vi "Sensor_Readings_Intg.vi"(0 "LINX Resource in":T1, 1 "Gyro Offset Y":i16, 2 "Gyro Offset X":i16, 3 "I2C Slave Address":T7, 4 "Milliseconds to wait in":u32=1, 5 "Acc Offset X":dbl[](array[numeric])=[30.0], 6 "Acc Offset Y":dbl[](array[numeric])=[90.0], 7 "error in (no error)":errorcluster) -> (20 "LINX Resource out":T1, 21 "Gyro Angle X":dbl(graph), 22 "Gyro Angle Y":dbl(graph), 23 "Milliseconds to wait out":u32=1, 24 "Acc Angle X":dbl[](graph)=[-22.25165725221299], 25 "Acc Angle Y":dbl[](graph)=[-0.6417100508007536], 27 "error out":errorcluster)   [LabVIEW 2021]
uses:
  <vilib>/MakerHub/LINX/Private/Type Defs/LINX Ref.ctl
  <vilib>/MakerHub/LINX/Private/Type Defs/Platform.ctl
  <vilib>/MakerHub/LINX/Private/Type Defs/Interface.ctl
  <vilib>/MakerHub/LINX/Private/Device/Type Defs/LINX Device Config.ctl
  <vilib>/MakerHub/LINX/Private/Device/Type Defs/TCP Config.ctl
  <vilib>/MakerHub/LINX/Private/Device/Type Defs/Channels.ctl
  <vilib>/MakerHub/LINX/Public/Sensors/Accelerometer/MPU60X0/DeviceAddresses.ctl
  <vilib>/MakerHub/LINX/Public/Sensors/Accelerometer/MPU60X0/MPU60X0.lvlib
  <vilib>/MakerHub/LINX/LMH-LINX.lvlib
  <vilib>/MakerHub/LINX/Private/Device/Device.lvlib
panel:
  out "Acceleration Graph":T8(graph)={"X Axis"=-7900, "Y Axis"=-136, "Z Axis"=-14032}
  out "Acceleration Data (g)":T8={"X Axis"=-7900, "Y Axis"=-136, "Z Axis"=-14032}
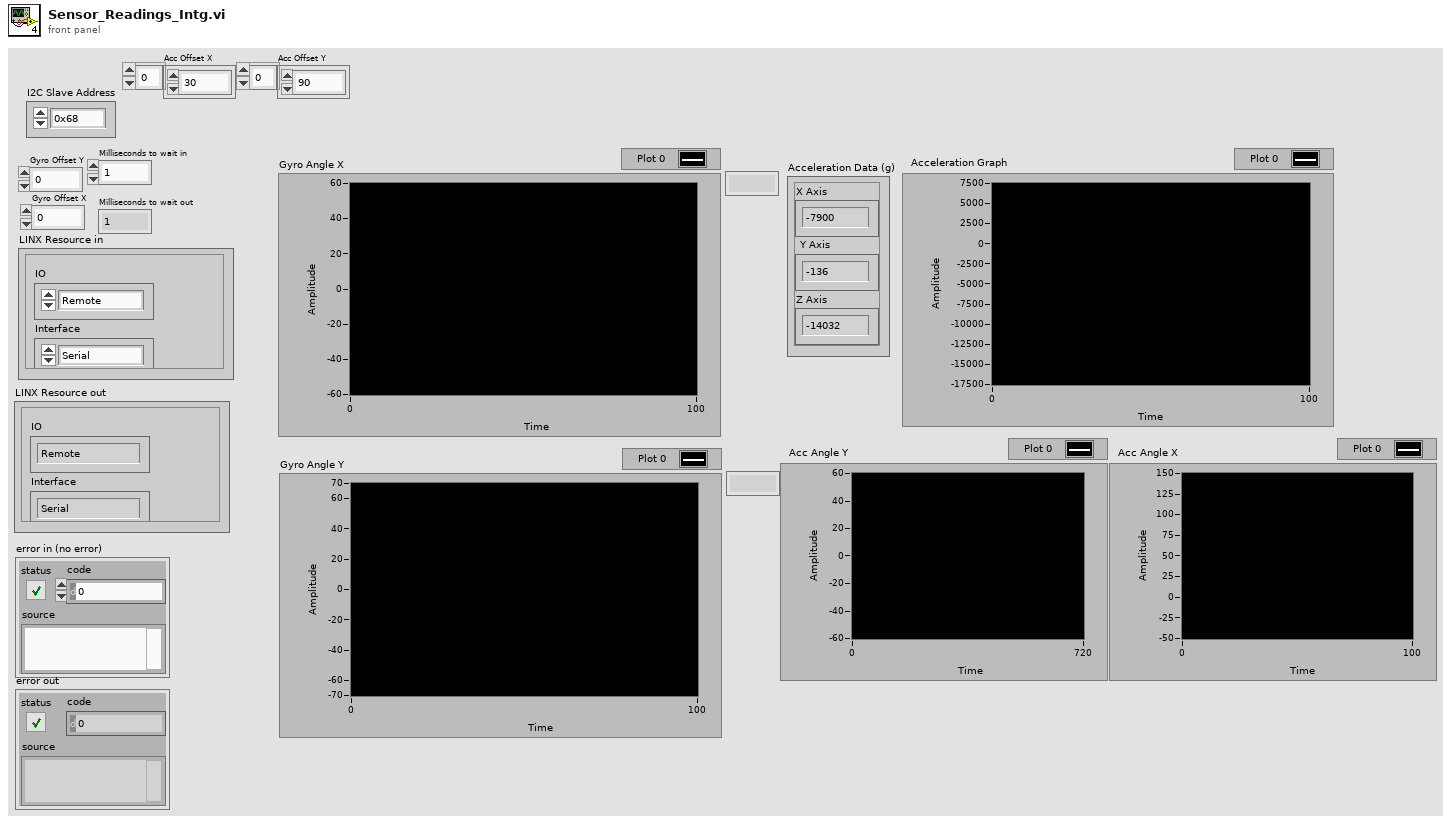
[diagram p1: front panel]
types:
  T1 = typedef "LMH-LINX.lvlib/LINX Ref.ctl" = cluster{"IO":T2, "Interface":T3, "LINX Device Config":T4}
  T2 = typedef "LMH-LINX.lvlib/Platform.ctl" = enum16{"Remote", "Local"}
  T3 = typedef "LMH-LINX.lvlib/Interface.ctl" = enum16{"Serial", "TCP"}
  T4 = typedef "LMH-LINX.lvlib/Device.lvlib/LINX Device Config.ctl" = cluster{"Interface":T3, "COM Port":refnum<visa-resource-name>, "TCP Configuration":T5, "Device Family":u8, "Device ID":u8, "Device Name":string, "TCP Ref":refnum<k5>, "Channels":T6}
  T5 = typedef "LMH-LINX.lvlib/Device.lvlib/TCP Config.ctl" = cluster{"IP Address":string, "Port":u16}
  T6 = typedef "LMH-LINX.lvlib/Channels.ctl" = cluster{"DI":u8[], "DO":u8[], "AI":u8[], "AO":u8[], "PWM":u8[], "QE":u8[], "UART":u8[], "I2C 2":u8[], "SPI":u8[], "CAN":u8[], "Servo":u8[], "AI Ref (V)":dbl, "AI Resolution (Bits)":u8, "AO Ref (V)":dbl, "AO Resolution (Bits)":u8}
  T7 = typedef "LMH-LINX.lvlib/MPU60X0.lvlib/DeviceAddresses.ctl" = enum16{"0x68", "0x69"}
  T8 = cluster{"X Axis":i16, "Y Axis":i16, "Z Axis":i16}
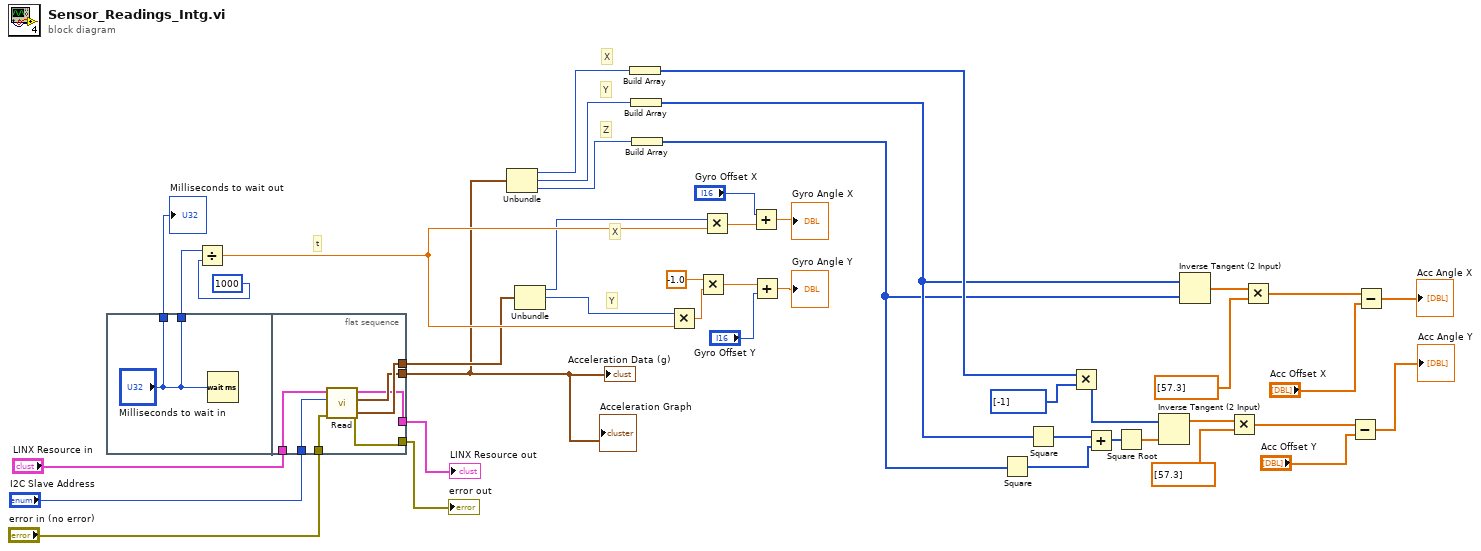
[diagram p0: block diagram]
diagram:
  # "Z"
  # "Y"
  # "X"
  # "X"
  # "Y"
  # "t"
  n1 = flat-sequence {
    tunnel: ["Milliseconds to wait in"] -> w41
    tunnel: ["Milliseconds to wait in"] -> w25
    tunnel: "error in (no error)" -> [w51]
    tunnel: "LINX Resource in" -> [w50]
    tunnel: [w49] -> w40
    tunnel: [w48] -> w4
    tunnel: [w47] -> w27
    tunnel: [w46] -> w26
    tunnel: "I2C Slave Address" -> [w45]
    frame #0 {
      n2 = Wait (ms)(milliseconds to wait="Milliseconds to wait in") -> ()  [unwired: 1 out]
    }
    frame #1 {
      n3 = call <vilib>:"Read.vi"("Error In"=w51, "I2C Slave Address"=w45, "LINX Resource"=w50) -> ("Error Out"=w46:errorcluster, "Gyro  Data (dps)"=w49:T8, "Acceleration Data (g)"=w48:T8, "LINX Resource"=w47:T1)  [unwired: 4 in, 1 out]
    }
  }
  n4 = Divide(x=w41, y=u32 1000) -> (x/y=w42:dbl)
  n5 = Unbundle(w4) -> ("X Axis"=w1:i16, "Y Axis"=w2:i16, "Z Axis"=w3:i16)
  n6 = Unbundle(w40) -> ("X Axis"=w35:i16, "Y Axis"=w5:i16)  [unwired: 1 out]
  n7 = Build Array(w1) -> (w22:i16[])
  n8 = Build Array(w2) -> (w19:i16[])
  n9 = Build Array(w3) -> (w18:i16[])
  n10 = Multiply(x=w5, y=w42) -> (x*y=w39:dbl)
  n11 = Multiply(x=-1.0, y=w39) -> (x*y=w29:dbl)
  n12 = Multiply(x=w35, y=w42) -> (x*y=w28:dbl)
  n13 = Add(x="Gyro Offset X", y=w28) -> (x+y=→"Gyro Angle X":dbl)
  n14 = Add(x=w29, y="Gyro Offset Y") -> (x+y=→"Gyro Angle Y":dbl)
  n15 = Square(x=w18) -> (x^2=w16:i16[])
  n16 = Square(x=w19) -> (x^2=w17:i16[])
  n17 = Multiply(x=w22, y=i16[] [-1]) -> (x*y=w21:i16[])
  n18 = Add(x=w17, y=w16) -> (x+y=w15:i16[])
  n19 = Square Root(x=w15) -> (sqrt(x)=w20:dbl[])
  n20 = Inverse Tangent (2 Input)(1:w20, 2:w21) -> (0:w13:dbl[])
  n21 = Inverse Tangent (2 Input)(1:w18, 2:w19) -> (0:w23:dbl[])
  n22 = Multiply(x=w13, y=dbl[] [57.3]) -> (x*y=w7:dbl[])
  n23 = Multiply(x=w23, y=dbl[] [57.3]) -> (x*y=w11:dbl[])
  n24 = Subtract(x=w7, y="Acc Offset Y") -> (x-y=→"Acc Angle Y":dbl[])
  n25 = Subtract(x=w11, y="Acc Offset X") -> (x-y=→"Acc Angle X":dbl[])
  "Acceleration Data (g)" <- w4
  "Acceleration Graph" <- w4
  "LINX Resource out" <- w27
  "error out" <- w26
  "Milliseconds to wait out" <- w25
